vi "VFH-read_folder-nanoVNA.vi"(10 "Folder Path":path) -> (0 "Data Points":i32, 1 "size(s)":i32, 2 "avg output":T1)   [LabVIEW 2020, in "VFH-VNA_File_Handler.lvlib"]
uses:
  VFH-VNA_File_Handler.lvlib
  VFH-file_cluster-NanoVNA.ctl
panel:
  out "Array":T1[](array[typedef])
  out "Array 5":dbl[][](array[numeric])
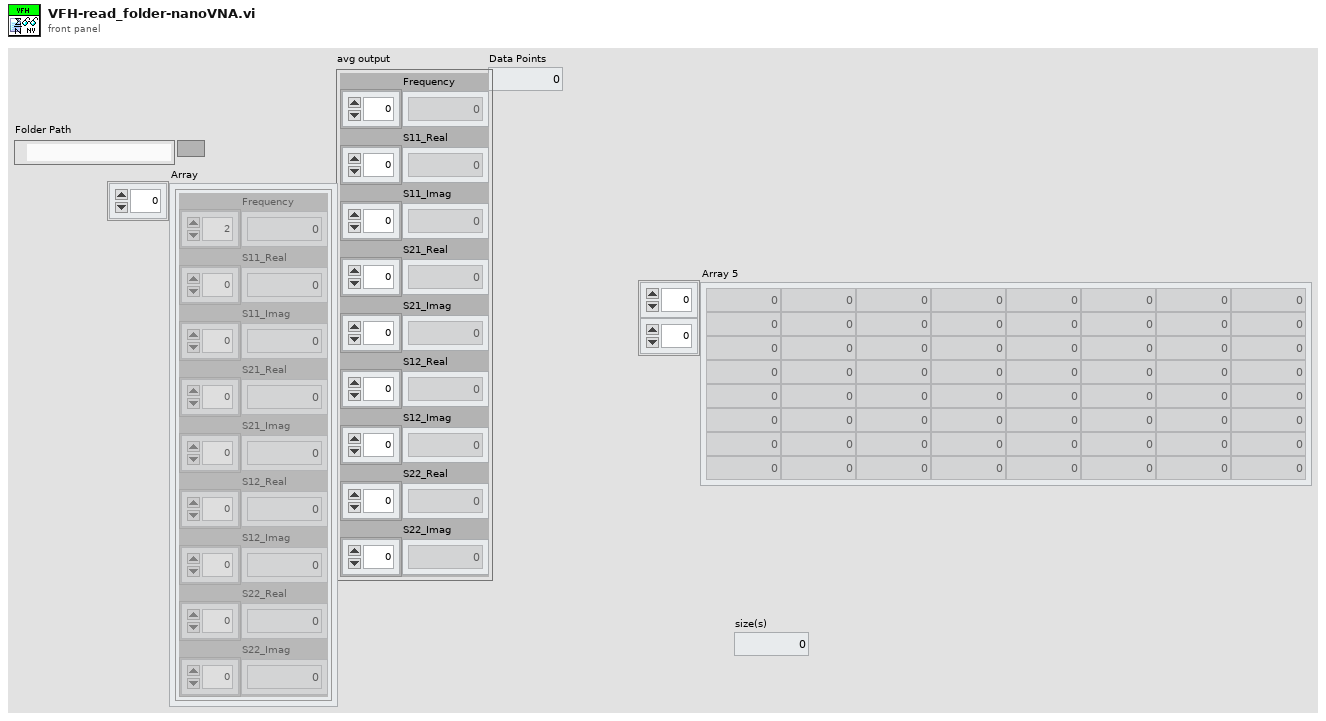
[diagram p1: front panel]
types:
  T1 = typedef "VFH-VNA_File_Handler.lvlib/VFH-file_cluster-NanoVNA.ctl" = cluster{"Frequency":dbl[], "S11_Real":dbl[], "S11_Imag":dbl[], "S21_Real":dbl[], "S21_Imag":dbl[], "S12_Real":dbl[], "S12_Imag":dbl[], "S22_Real":dbl[], "S22_Imag":dbl[]}
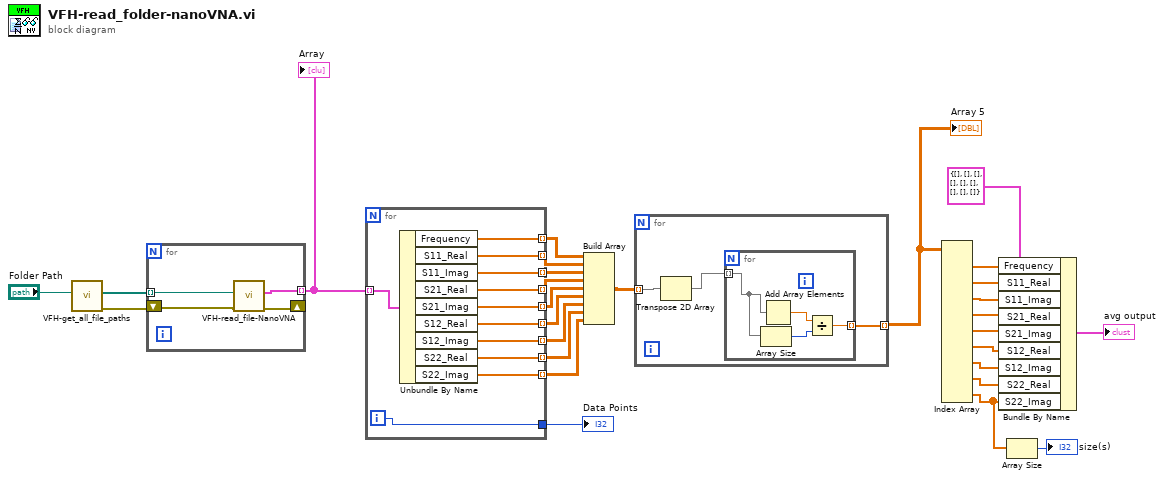
[diagram p0: block diagram]
diagram:
  n1 = call "VFH-get_all_file_paths.vi"("Folder Path"="Folder Path") -> ("error out"=w27:errorcluster, "All Files in Dir"=w26:path[])  [unwired: 8 in, 1 out]
  n2 = for {
    shift-right: [w29] -> _
    shift-left: w27 -> [w30]
    tunnel: w26 -> [w32] mode=indexing
    tunnel: [w31] -> w25 mode=indexing
    n3 = call "VFH-read_file-NanoVNA.vi"("error in"=w30, "file path (dialog if empty)"=w32) -> ("error out"=w29:errorcluster, "output cluster"=w31:T1)  [unwired: 8 in]
  }
  "Array" <- w25
  n4 = for {
    tunnel: w25 -> [w43] mode=indexing
    tunnel: [w42] -> w24 mode=indexing
    tunnel: [w41] -> w23 mode=indexing
    tunnel: [w40] -> w22 mode=indexing
    tunnel: [w39] -> w21 mode=indexing
    tunnel: [w38] -> w20 mode=indexing
    tunnel: [w37] -> w19 mode=indexing
    tunnel: [w36] -> w18 mode=indexing
    tunnel: [w35] -> w15 mode=indexing
    tunnel: [w34] -> w14 mode=indexing
    tunnel: [w33] -> w1
    i -> [w33]
    n5 = Unbundle By Name(w43) -> ("Frequency"=w42:dbl[], "S11_Real"=w41:dbl[], "S11_Imag"=w40:dbl[], "S21_Real"=w39:dbl[], "S21_Imag"=w38:dbl[], "S12_Real"=w37:dbl[], "S12_Imag"=w36:dbl[], "S22_Real"=w35:dbl[], "S22_Imag"=w34:dbl[])
  }
  "Data Points" <- w1
  n6 = Build Array(w24, w23, w22, w21, w20, w19, w18, w15, w14) -> (w17:dbl[][][])
  n7 = for {
    tunnel: w17 -> [w46] mode=indexing
    tunnel: [w44] -> w16 mode=indexing
    n8 = Transpose 2D Array(2D array=w46) -> (transposed array=w45:dbl[][])
    n9 = for {
      tunnel: w45 -> [w48] mode=indexing
      tunnel: [w47] -> w44 mode=indexing
      n10 = Array Size(array=w48) -> (size(s)=w50:i32)
      n11 = Add Array Elements(numeric array=w48) -> (sum=w49:dbl)
      n12 = Divide(x=w49, y=w50) -> (x/y=w47:dbl)
    }
  }
  "Array 5" <- w16
  n13 = Index Array(array=w16) -> (element #1=w11:dbl[], element #2=w10:dbl[], element #3=w9:dbl[], element #4=w8:dbl[], element #5=w7:dbl[], element #6=w6:dbl[], element #7=w5:dbl[], element #8=w4:dbl[], element #9=w3:dbl[])  [unwired: 18 in]
  n14 = Bundle By Name(cluster=T1 {"Frequency"=[], "S11_Real"=[], "S11_Imag"=[], "S21_Real"=[], "S21_Imag"=[], "S12_Real"=[], "S12_Imag"=[], "S22_Real"=[], "S22_Imag"=[]} ("output cluster"), "Frequency"=w11, "S11_Real"=w10, "S11_Imag"=w9, "S21_Real"=w8, "S21_Imag"=w7, "S12_Real"=w6, "S12_Imag"=w5, "S22_Real"=w4, "S22_Imag"=w3) -> (→"avg output":T1)
  n15 = Array Size(array=w3) -> (size(s)=→"size(s)":i32)
